vi "Vin_Vout_Calc.vi"(0 "aDATA":u8[](array[numeric])) -> (1 "CH R":u8, 2 "V in":dbl, 3 "V Out":dbl)   [LabVIEW 2010]
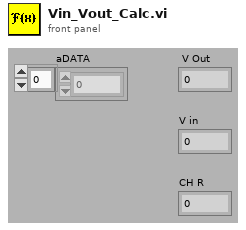
[diagram p1: front panel]
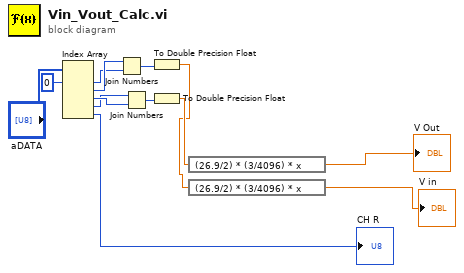
[diagram p0: block diagram]
diagram:
  n1 = Index Array(array="aDATA", index #1=0 ("index")) -> (element #1=w9:u8, element #2=w10:u8, element #3=w12:u8, element #4=w11:u8, element #5=→"CH R":u8)  [unwired: 4 in]
  n2 = Join Numbers(hi=w10, lo=w9) -> ((hi.lo)=w6:u16)
  n3 = Join Numbers(hi=w11, lo=w12) -> ((hi.lo)=w5:u16)
  n4 = To Double Precision Float(number=w6) -> (double precision float=w3:dbl)
  n5 = To Double Precision Float(number=w5) -> (double precision float=w4:dbl)
  n6 = expression code="(26.9/2) * (3/4096) * x"(w4) -> (→"V Out":dbl)
  n7 = expression code="(26.9/2) * (3/4096) * x"(w3) -> (→"V in":dbl)
